vi "Gear Aiming v2.vi"() -> (2 "Drive Rotate":dbl, 3 "Drive Y":dbl)   [LabVIEW 2016]
uses:
  <vilib>/Rock Robotics/Network Tables/NT Read Numeric Array.vi
  Robot Global Data.vi
panel:
  in  "PID gains":T1={"proportional gain (Kc)"=0.019, "integral time (Ti, min)"=0.0, "derivative time (Td, min)"=0.0} {"derivative time (Td, min)" format="%.3f"; "integral time (Ti, min)" format="%.3f"; "proportional gain (Kc)" format="%.3f"}
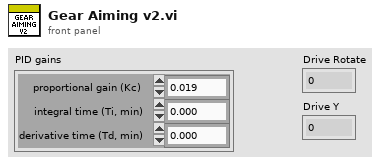
[diagram p1: front panel]
types:
  T1 = cluster{"proportional gain (Kc)":dbl, "integral time (Ti, min)":dbl, "derivative time (Td, min)":dbl}
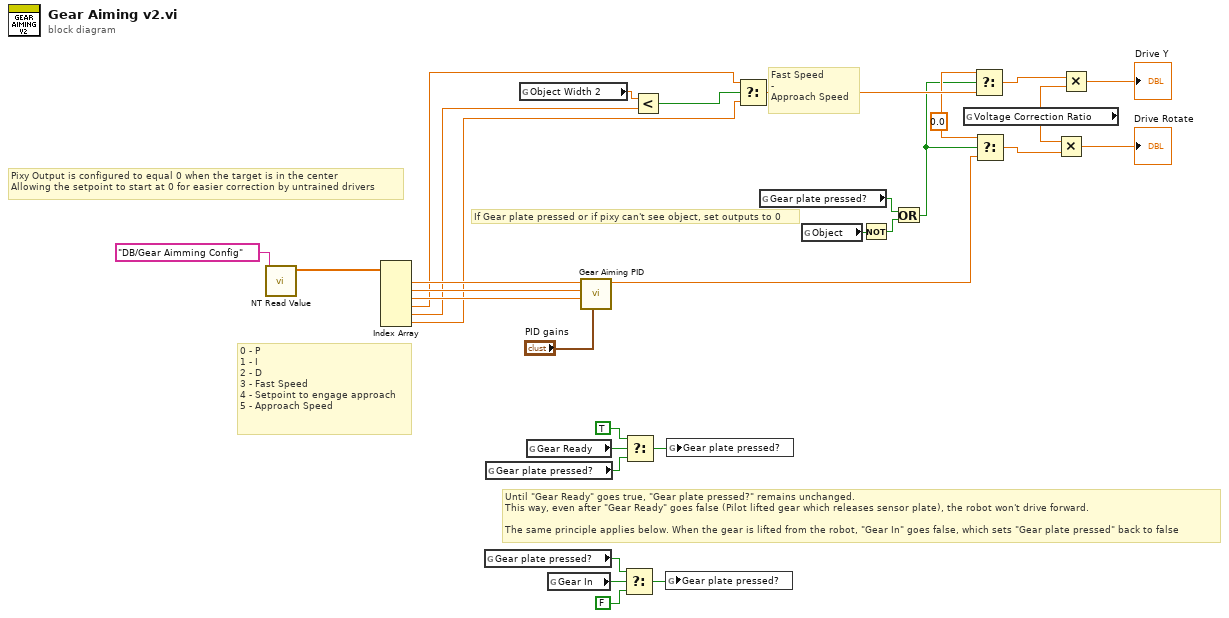
[diagram p0: block diagram]
diagram:
  w28 = 0.0 ("t")
  # "Pixy Output is configured to equal 0 when the target is in the center\nAllowing the setpoint to start at 0 for easier correction by untrained drivers"
  # "0 - P\n1 - I\n2 - D\n3 - Fast Speed\n4 - Setpoint to engage approach\n5 - Approach Speed"
  # "Fast Speed\n-\nApproach Speed"
  # "Until \"Gear Ready\" goes true, \"Gear plate pressed?\" remains unchanged.\nThis way, even after \"Gear Ready\" goes false (Pilot lifted gear which releases sensor plate), the robot won't drive forward.\n\nThe same principle applies below. When the gear is lifted from the robot, \"Gear In\" goes false, which sets \"Gear plate pressed\" back to false"
  # "If Gear plate pressed or if pixy can't see object, set outputs to 0"
  n1 = call-poly <vilib>:"NT Read Value.vi"("Name"="DB/Gear Aimming Config") -> ("Numeric Array"=w16:dbl[])  [unwired: 9 in, 1 out]
  n2 = Index Array(array=w16) -> (element #1=w14:dbl, element #2=w13:dbl, element #3=w12:dbl, element #4=w10:dbl, element #5=w9:dbl, element #6=w11:dbl)  [unwired: 6 in]
  n3 = global read "Robot Global Data.vi" "Gear plate pressed?"() -> (w18:bool)
  n4 = global read "Robot Global Data.vi" "Gear plate pressed?"() -> (w22:bool)
  n5 = global read "Robot Global Data.vi" "Object Width 2"() -> (w7:dbl)
  n6 = global read "Robot Global Data.vi" "Gear Ready"() -> (w25:bool)
  n7 = global read "Robot Global Data.vi" "Gear In"() -> (w21:bool)
  n8 = call "Gear Aiming PID.vi"("PID gains"="PID gains", "D"=w12, "I"=w13, "P"=w14) -> ("output"=w29:dbl)  [unwired: 7 in]
  n9 = Select(t=w18, s=w21, f=FALSE) -> (s? t:f=w20:bool)
  n10 = Select(t=TRUE, s=w25, f=w22) -> (s? t:f=w23:bool)
  n11 = Less?(x=w7, y=w9) -> (x < y?=w6:bool)
  n12 = global write "Robot Global Data.vi" "Gear plate pressed?"(w20) -> ()
  n13 = global write "Robot Global Data.vi" "Gear plate pressed?"(w23) -> ()
  n14 = Select(t=w10, s=w6, f=w11) -> (s? t:f=w31:dbl)
  n15 = global read "Robot Global Data.vi" "Gear plate pressed?"() -> (w26:bool)
  n16 = global read "Robot Global Data.vi" "Object"() -> (w27:bool)
  n17 = Not(x=w27) -> (.not. x?=w1:bool)
  n18 = Or(x=w26, y=w1) -> (x .or. y?=w8:bool)
  n19 = global read "Robot Global Data.vi" "Voltage Correction Ratio"() -> (w2:dbl)
  n20 = Select(t=w28, s=w8, f=w31) -> (s? t:f=w3:dbl)
  n21 = Select(t=w28, s=w8, f=w29) -> (s? t:f=w30:dbl)
  n22 = Multiply(x=w2, y=w30) -> (x*y=→"Drive Rotate":dbl)
  n23 = Multiply(x=w3, y=w2) -> (x*y=→"Drive Y":dbl)
